vi "Prueba 4 Lester Roche.vi"() -> ()   [LabVIEW 2011]
uses:
  ControlPrueba4 Lester Roche.ctl
panel:
  out "Array":T1(array[cluster]) {"Tanque 4" scale=0.0..60.0; "Tanque 3" scale=0.0..60.0; "Tanque 2" scale=0.0..60.0; "Tanque 1" scale=0.0..60.0}
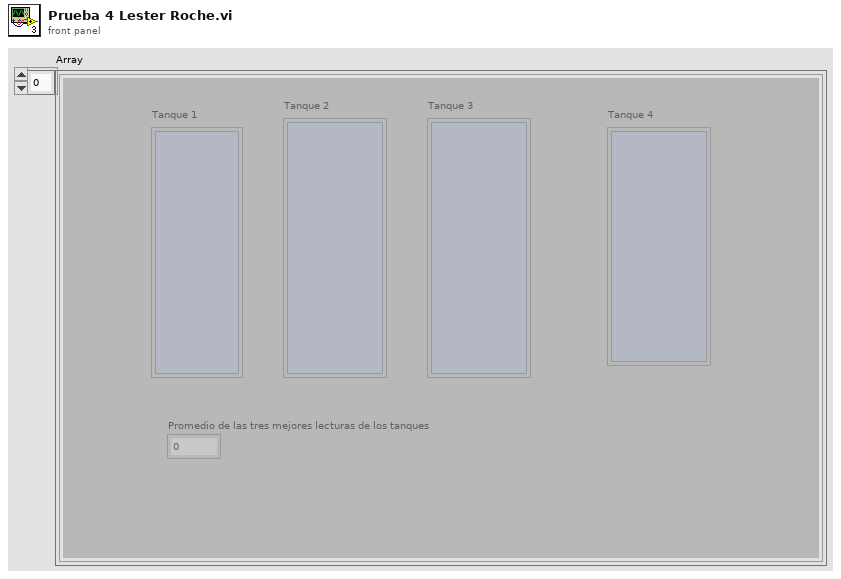
[diagram p1: front panel]
types:
  T1 = cluster{"Tanque 1":i32, "Tanque 2":i32, "Tanque 3":i32, "Tanque 4":i32, "Promedio de las tres mejores lecturas de los tanques":dbl}[]
  T2 = typedef "ControlPrueba4 Lester Roche.ctl" = enum16{"Inicialiazar variables", "rellenar tanques", "promedio de las tres mejores lecturas", "finalizar"}
  T3 = cluster{"Tanque 1":i32, "Tanque 2":i32, "Tanque 3":i32, "Tanque 4":i32, "Promedio de las tres mejores lecturas de los tanques":dbl}
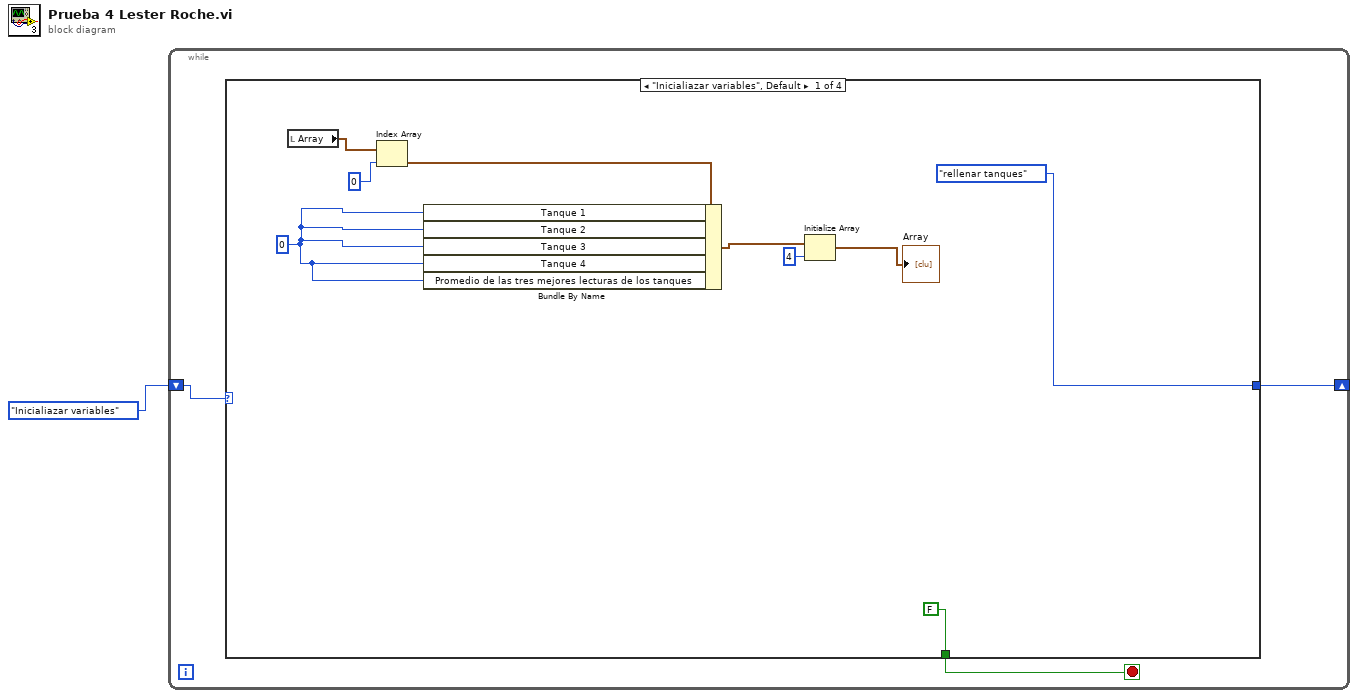
[diagram p0: block diagram]
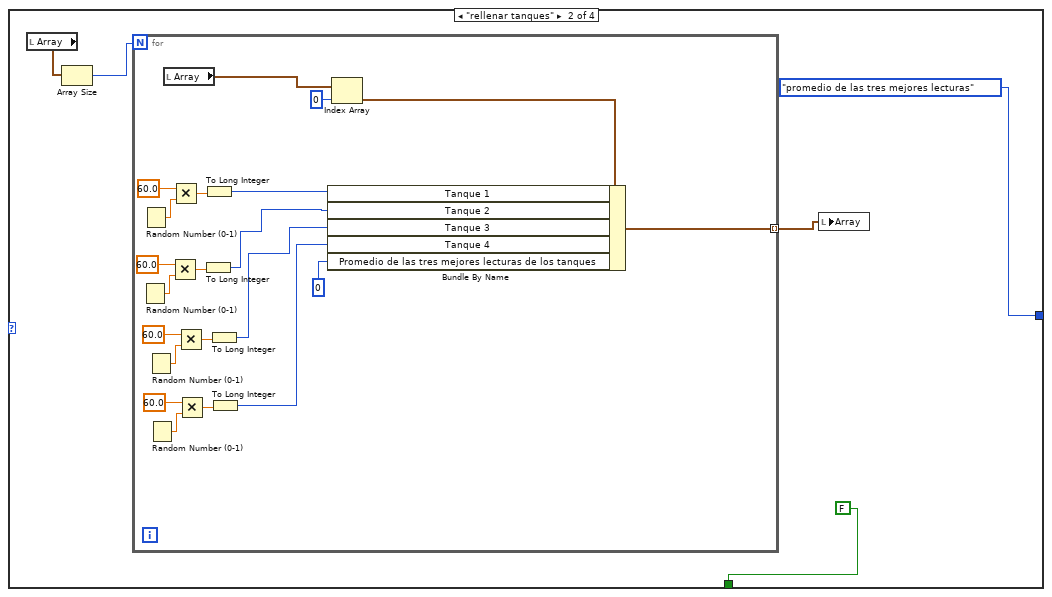
[diagram p2: hidden frame]
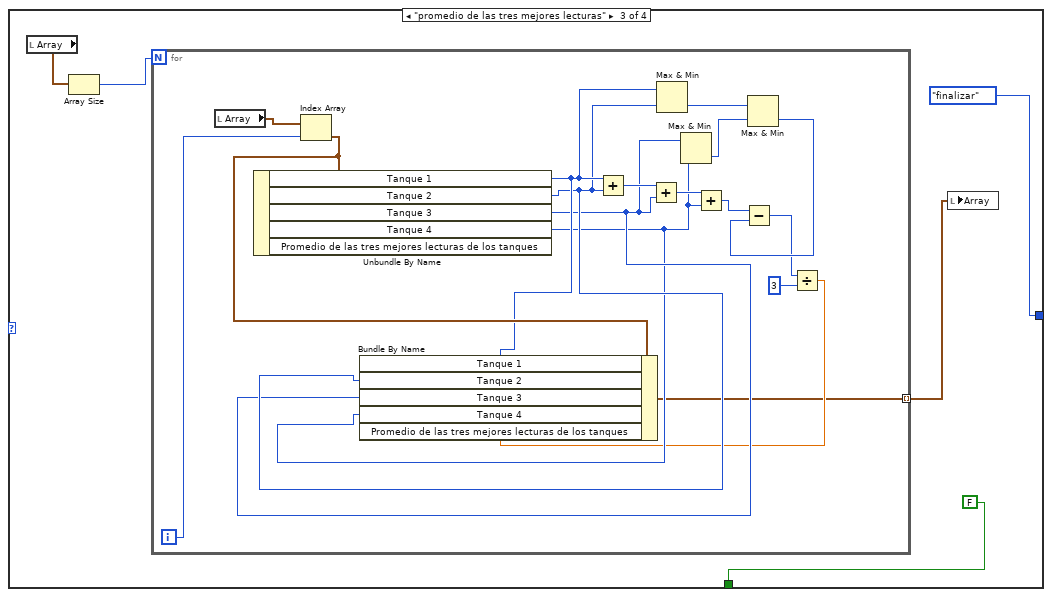
[diagram p3: hidden frame]
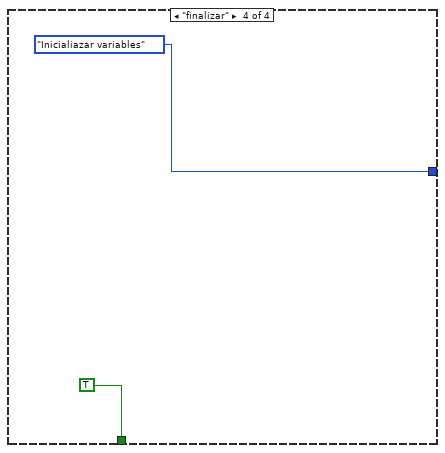
[diagram p4: hidden frame]
diagram:
  n1 = while {
    shift-right: [w3] -> _
    shift-left: ControlPrueba4_Lester_Roche."Inicialiazar variables" -> [w4]
    stop <- w2 stop-if-true
    n2 = case shown="\"Inicialiazar variables\", Default" w4 {
      tunnel: [ControlPrueba4_Lester_Roche."rellenar tanques" ControlPrueba4_Lester_Roche."promedio de las tres mejores lecturas" ControlPrueba4_Lester_Roche."finalizar" ControlPrueba4_Lester_Roche."Inicialiazar variables"] -> w3
      tunnel: [FALSE FALSE FALSE TRUE] -> w2
      frame "Inicialiazar variables", Default {
        w10 = 0
        n3 = local read "Array"() -> (w13:T1)
        n4 = Index Array(array=w13, index=0) -> (element=w11:T3)
        n5 = Bundle By Name(cluster=w11, "Tanque 1"=w10, "Tanque 2"=w10, "Tanque 3"=w10, "Tanque 4"=w10, "Promedio de las tres mejores lecturas de los tanques"=w10) -> (w9:T3)
        n6 = Initialize Array(w9, 4 ("dimension size")) -> (→"Array":T1)
      }
      frame "rellenar tanques" {
        n7 = local read "Array"() -> (w18:T1)
        n8 = Array Size(array=w18) -> (size(s)=w17:i32)
        n9 = for {
          N: w17 -> [_]
          tunnel: [w19] -> w16 mode=indexing
          n10 = Random Number (0-1)() -> (number: 0 to 1=w31:dbl)
          n11 = Random Number (0-1)() -> (number: 0 to 1=w35:dbl)
          n12 = Random Number (0-1)() -> (number: 0 to 1=w27:dbl)
          n13 = Random Number (0-1)() -> (number: 0 to 1=w24:dbl)
          n14 = local read "Array"() -> (w39:T1)
          n15 = Multiply(x=60.0, y=w31) -> (x*y=w32:dbl)
          n16 = Multiply(x=60.0, y=w35) -> (x*y=w34:dbl)
          n17 = Multiply(x=60.0, y=w27) -> (x*y=w26:dbl)
          n18 = Multiply(x=60.0, y=w24) -> (x*y=w25:dbl)
          n19 = To Long Integer(number=w32) -> (32bit integer=w29:i32)
          n20 = To Long Integer(number=w34) -> (32bit integer=w33:i32)
          n21 = To Long Integer(number=w26) -> (32bit integer=w22:i32)
          n22 = To Long Integer(number=w25) -> (32bit integer=w21:i32)
          n23 = Index Array(array=w39, index=0) -> (element=w37:T3)
          n24 = Bundle By Name(cluster=w37, "Tanque 1"=w33, "Tanque 2"=w29, "Tanque 3"=w22, "Tanque 4"=w21, "Promedio de las tres mejores lecturas de los tanques"=0) -> (w19:T3)
        }
        n25 = local write "Array"(w16) -> ()
      }
      frame "promedio de las tres mejores lecturas" {
        n26 = local read "Array"() -> (w44:T1)
        n27 = Array Size(array=w44) -> (size(s)=w43:i32)
        n28 = for {
          N: w43 -> [_]
          tunnel: [w45] -> w42 mode=indexing
          i -> [w60]
          n29 = local read "Array"() -> (w61:T1)
          n30 = Index Array(array=w61, index=w60) -> (element=w53:T3)
          n31 = Unbundle By Name(w53) -> ("Tanque 1"=w52:i32, "Tanque 2"=w51:i32, "Tanque 3"=w50:i32, "Tanque 4"=w49:i32)  [unwired: 1 out]
          n32 = Add(x=w52, y=w51) -> (x+y=w59:i32)
          n33 = Add(x=w59, y=w50) -> (x+y=w58:i32)
          n34 = Max & Min(x=w52, y=w51) -> (min(x,y)=w56:i32)  [unwired: 1 out]
          n35 = Max & Min(x=w50, y=w49) -> (min(x,y)=w55:i32)  [unwired: 1 out]
          n36 = Add(x=w58, y=w49) -> (x+y=w57:i32)
          n37 = Max & Min(x=w56, y=w55) -> (min(x,y)=w54:i32)  [unwired: 1 out]
          n38 = Subtract(x=w57, y=w54) -> (x-y=w48:i32)
          n39 = Divide(x=w48, y=3) -> (x/y=w46:dbl)
          n40 = Bundle By Name(cluster=w53, "Tanque 1"=w52, "Tanque 2"=w51, "Tanque 3"=w50, "Tanque 4"=w49, "Promedio de las tres mejores lecturas de los tanques"=w46) -> (w45:T3)
        }
        n41 = local write "Array"(w42) -> ()
      }
      frame "finalizar" {
      }
    }
  }
